vi "similiraty_cleaning.vi"(8 "error in (no error)":errorcluster, 9 "I channel in":cluster{"BG":sgl[], "Ie":sgl[], "I0":sgl[]}[](array[cluster]), 10 "II channel in":cluster{"BG":sgl[], "Ie":sgl[], "I0":sgl[]}[](array[cluster]), 11 "Detector in":refnum<class "Detector.lvclass">) -> (0 "error out":errorcluster, 1 "II channel out":cluster{"BG":sgl[], "Ie":sgl[], "I0":sgl[]}[](array[cluster]), 2 "I channel out":cluster{"BG":sgl[], "Ie":sgl[], "I0":sgl[]}[](array[cluster]), 3 "Detector out":refnum<class "Detector.lvclass">)   [LabVIEW 2020, in "Detector.lvclass"]
uses:
  Detector.lvclass
  Detector.lvclass/Detector.ctl
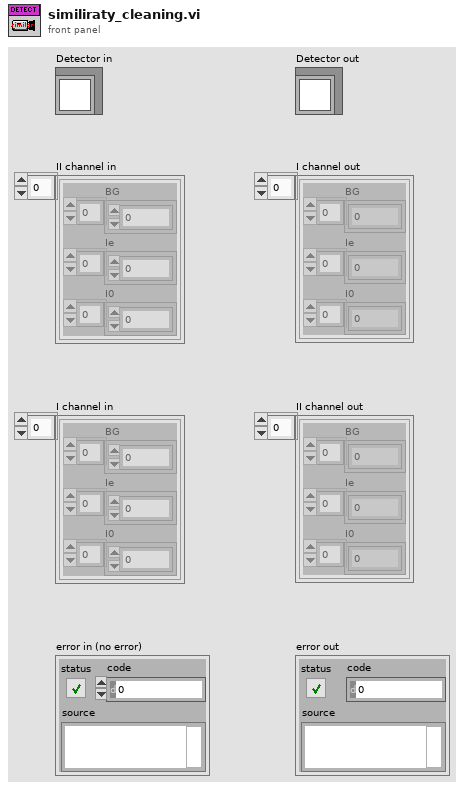
[diagram p1: front panel]
types:
  T1 = typedef "Control-Client.lvclass/Controls-refs_CLIENT.ctl" = cluster{"ON/OFF Cool":refnum<vi>, "Save spectra":refnum<vi>, "Read detector":refnum<vi>, "# scans":refnum<vi>, "BG-level":refnum<vi>, "Set T":refnum<vi>, "Termometer":refnum<vi>, "Spectra":refnum<vi>, "Error Meter_ref":refnum<vi>, "OD graph":refnum<vi>, "from_pixel":refnum<vi>, "to_pixel":refnum<vi>, "threshold_ref_channel":refnum<vi>, "value":refnum<vi>, "python session":refnum<vi>, "ref h5_file":T2, "distance":refnum<vi>}
  T2 = typedef "hid_t.ctl" = i64
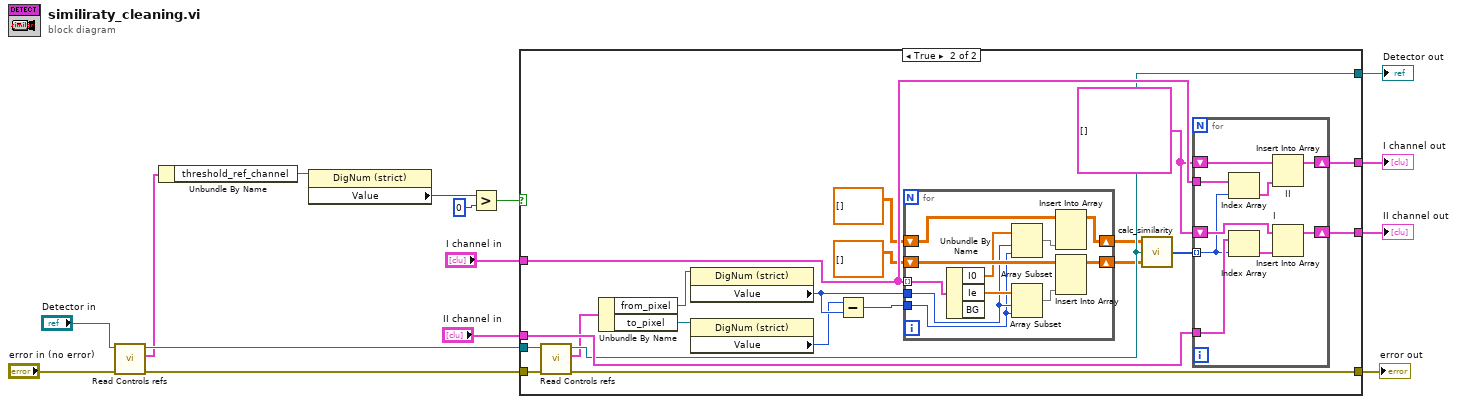
[diagram p0: block diagram]
diagram:
  n1 = call "Read Controls refs.vi"("error in (no error)"="error in (no error)", "Detector in"="Detector in") -> ("error out"=w2:errorcluster, "Controls refs"=w7:T1, "Detector out"=w9:refnum<class "Detector.lvclass">)  [unwired: 7 in]
  n2 = Unbundle By Name(w7) -> ("threshold_ref_channel"=w8:refnum<vi>)
  n3 = property class="DigNum (strict)"(reference=w8) -> ("Value"=w13:i32)  [unwired: 1 in, 2 out]
  n4 = Greater?(x=w13, y=0) -> (0:w11:bool)
  n5 = case shown="True" w11 {
    tunnel: [w19 w37] -> w4
    tunnel: "I channel in" -> [w19 w39]
    tunnel: "II channel in" -> [w18 w38]
    tunnel: [w18 w36] -> w3
    tunnel: w9 -> [w17 w35]
    tunnel: [w17 w34] -> w12
    tunnel: w2 -> [w16 w21]
    tunnel: [w16 w20] -> w1
    frame False {
    }
    frame True {
      w30 = cluster{"BG":sgl[], "Ie":sgl[], "I0":sgl[]}[] [] ("I channel")
      n6 = call "Read Controls refs.vi"("error in (no error)"=w21, "Detector in"=w35) -> ("error out"=w20:errorcluster, "Controls refs"=w26:T1, "Detector out"=w34:refnum<class "Detector.lvclass">)  [unwired: 7 in]
      n7 = Unbundle By Name(w26) -> ("from_pixel"=w25:refnum<vi>, "to_pixel"=w24:refnum<vi>)
      n8 = property class="DigNum (strict)"(reference=w25) -> ("Value"=w23:i32)  [unwired: 1 in, 2 out]
      n9 = property class="DigNum (strict)"(reference=w24) -> ("Value"=w22:i32)  [unwired: 1 in, 2 out]
      n10 = Subtract(x=w22, y=w23) -> (x-y=w27:i32)
      n11 = for {
        tunnel: w39 -> [w59] mode=indexing
        shift-right: [w57] -> w31
        shift-left: dbl[][] [] -> [w58]
        shift-right: [w55] -> w28
        shift-left: dbl[][] [] -> [w56]
        tunnel: w23 -> [w50]
        tunnel: w27 -> [w49]
        n12 = Unbundle By Name(w59) -> ("I0"=w52:sgl[], "Ie"=w54:sgl[])  [unwired: 1 out]
        n13 = Array Subset(array=w52, index=w50, length=w49) -> (w51:sgl[])
        n14 = Array Subset(array=w54, index=w50, length=w49) -> (w53:sgl[])
        n15 = Insert Into Array(array=w58, new element=w51) -> (w57:dbl[][])  [unwired: 2 in]
        n16 = Insert Into Array(array=w56, new element=w53) -> (w55:dbl[][])  [unwired: 2 in]
      }
      n17 = call "calc_similarity.vi"("data2"=w28, "Detector in"=w34, "data1"=w31) -> ("similarity out"=w29:i32[])
      n18 = for {
        tunnel: w38 -> [w48]
        shift-right: [w45] -> w36
        shift-left: w30 -> [w46]
        shift-right: [w44] -> w37
        shift-left: w30 -> [w43]
        tunnel: w39 -> [w42]
        tunnel: w29 -> [w40] mode=indexing
        n19 = Index Array(array=w42, index=w40) -> (element=w41:cluster{"BG":sgl[], "Ie":sgl[], "I0":sgl[]})
        n20 = Index Array(array=w48, index=w40) -> (element=w47:cluster{"BG":sgl[], "Ie":sgl[], "I0":sgl[]})
        n21 = Insert Into Array "II"(array=w43, new element=w41) -> (w44:cluster{"BG":sgl[], "Ie":sgl[], "I0":sgl[]}[])  [unwired: 1 in]
        n22 = Insert Into Array "I"(array=w46, new element=w47) -> (w45:cluster{"BG":sgl[], "Ie":sgl[], "I0":sgl[]}[])  [unwired: 1 in]
      }
    }
  }
  "Detector out" <- w12
  "error out" <- w1
  "I channel out" <- w4
  "II channel out" <- w3
